vi "Blinking Lights.vi"() -> ()   [LabVIEW 2015]
panel:
  in  "stop":bool
  out "4":bool
  out "3":bool
  out "2":bool
  out "1":bool
  out "0":bool
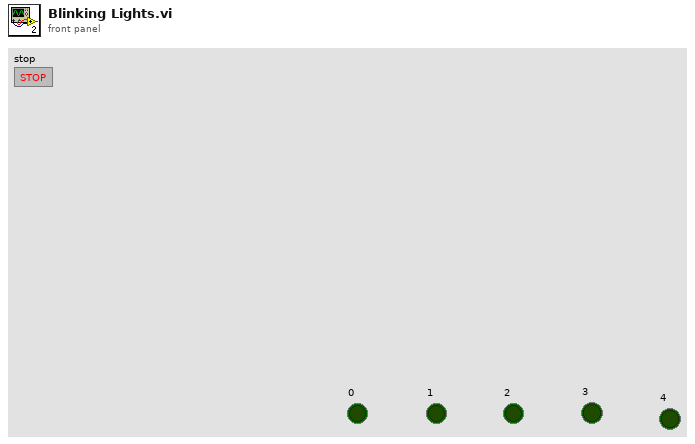
[diagram p1: front panel]
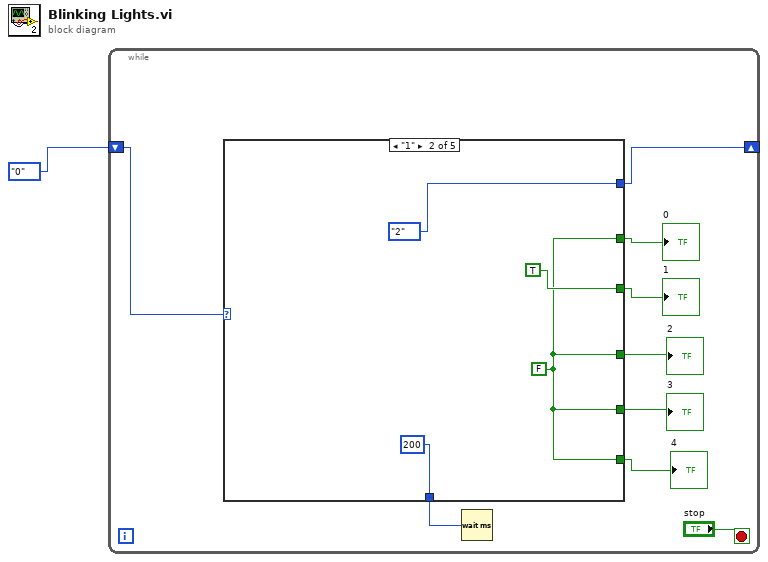
[diagram p0: block diagram]
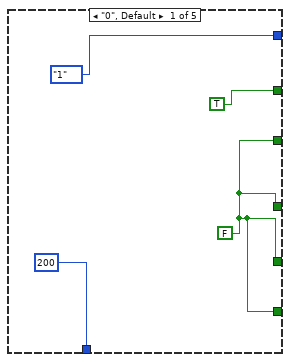
[diagram p2: hidden frame]
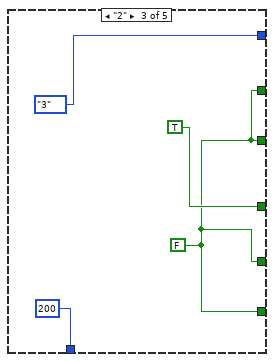
[diagram p3: hidden frame]
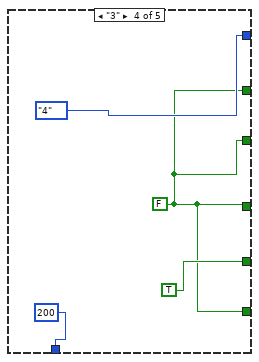
[diagram p4: hidden frame]
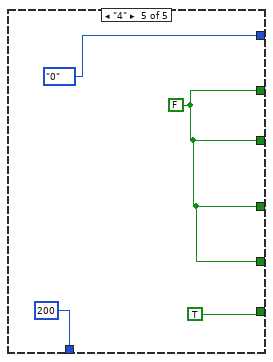
[diagram p5: hidden frame]
diagram:
  n1 = while {
    shift-right: [w9] -> _
    shift-left: enum16{"0", "1", "2", "3", "4"}."0" -> [w10]
    stop <- "stop" stop-if-true
    n2 = case shown="\"1\"" w10 {
      tunnel: [enum16{"0", "1", "2", "3", "4"}."1" enum16{"0", "1", "2", "3", "4"}."2" enum16{"0", "1", "2", "3", "4"}."3" enum16{"0", "1", "2", "3", "4"}."4" enum16{"0", "1", "2", "3", "4"}."0"] -> w9
      tunnel: [TRUE w16 w20 w24 w28] -> w8
      tunnel: [w12 TRUE w20 w24 w28] -> w3
      tunnel: [w12 w16 TRUE w24 w28] -> w7
      tunnel: [w12 w16 w20 TRUE w28] -> w6
      tunnel: [w12 w16 w20 w24 TRUE] -> w5
      tunnel: [200 200 200 200 200] -> w4
      frame "0", Default {
        w12 = FALSE
      }
      frame "1" {
        w16 = FALSE
      }
      frame "2" {
        w20 = FALSE
      }
      frame "3" {
        w24 = FALSE
      }
      frame "4" {
        w28 = FALSE
      }
    }
    "0" <- w8
    "1" <- w3
    "2" <- w7
    "3" <- w6
    "4" <- w5
    n3 = Wait (ms)(milliseconds to wait=w4) -> ()  [unwired: 1 out]
  }
